vi "Intake Handler.vi"(11 "JoystickDevRef":T1) -> ()   [LabVIEW 2019]
uses:
  <vilib>/Rock Robotics/WPI/Joystick/WPI_JoystickDevRef.ctl
  <vilib>/Rock Robotics/WPI/Joystick/WPI_JoystickDeviceEnum.ctl
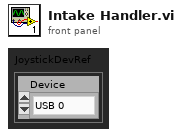
[diagram p1: front panel]
types:
  T1 = typedef "WPI_JoystickDevRef.ctl" = cluster{"Device":T2}
  T2 = typedef "WPI_JoystickDeviceEnum.ctl" = enum16{"USB 0", "USB 1", "USB 2", "USB 3", "USB 4", "USB 5"}
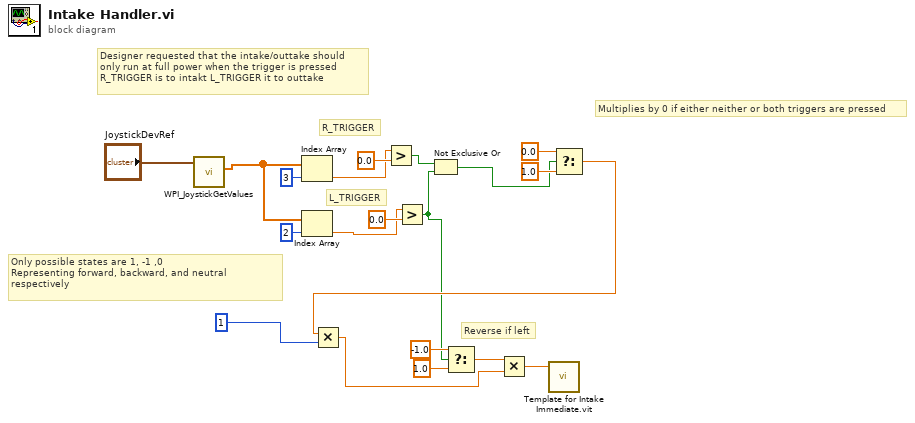
[diagram p0: block diagram]
diagram:
  # "Reverse if left"
  # "Multiplies by 0 if either neither or both triggers are pressed"
  # "Only possible states are 1, -1 ,0\nRepresenting forward, backward, and neutral respectively"
  # "Designer requested that the intake/outtake should \nonly run at full power when the trigger is pressed\nR_TRIGGER is to intakt L_TRIGGER it to outtake"
  # "R_TRIGGER"
  # "L_TRIGGER"
  n1 = call <vilib>:"WPI_JoystickGetValues.vi"("JoystickDevRef"="JoystickDevRef") -> ("Axes"=w19:dbl[])  [unwired: 6 in, 4 out]
  n2 = Index Array(array=w19, index=3) -> (element=w14:dbl)
  n3 = Index Array(array=w19, index=2) -> (element=w13:dbl)
  n4 = Greater?(x=w14, y=0.0) -> (0:w3:bool)
  n5 = Greater?(x=w13, y=0.0) -> (0:w1:bool)
  n6 = Not Exclusive Or(1:w1, 2:w3) -> (0:w2:bool)
  n7 = Select(t=-1.0, s=w1, f=1.0) -> (s? t:f=w8:dbl)
  n8 = Select(t=0.0, s=w2, f=1.0) -> (s? t:f=w12:dbl)
  n9 = Multiply(x=w12, y=1) -> (x*y=w7:dbl)
  n10 = Multiply(x=w8, y=w7) -> (x*y=w4:dbl)
  n11 = call "Template for Intake Immediate.vit"("Setpoint"=w4) -> ()  [unwired: 10 in, 1 out]
